vi "Read DO Data Value.vi"(8 "error in (no error)":errorcluster, 9 "Name":string, 10 "DO IOName (enum)":variant, 11 "DAQ":refnum<class "DAQ.lvclass">) -> (0 "error out":errorcluster, 2 "state":bool, 3 "DAQ":refnum<class "DAQ.lvclass">)   [LabVIEW 2017, in "DAQ.lvclass"]
doc: "Developed by Kevin Thompson\nkevin@thompsonengineering.net\n\nCopyright 2018-2020\nThompson Engineering, LLC"
uses:
  DAQ.lvclass
  DAQ.lvclass/DAQ.ctl
  <vilib>/DAQmx/read.llb/DAQmx Read (Digital Bool 1Line 1Point).vi
  Accessors/Get DAQ Settings.vi
  <vilib>/DAQmx/miscellaneous.llb/DAQmx Fill In Error Info.vi
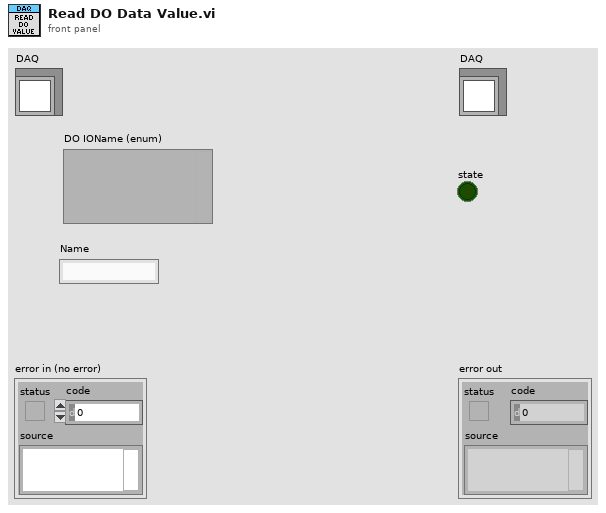
[diagram p1: front panel]
types:
  T1 = typedef "DAQ.lvclass/TD DAQ Settings--cluster.ctl" = cluster{"Simulate DAQ":bool, "DI Settings":T2[], "AI Settings":T3[], "Relay IONames":string[], "AO IONames":string[], "AO NChan SingleTask":bool}
  T2 = typedef "DAQ.lvclass/TD DI Instrument Settings--cluster.ctl" = cluster{"Disable":bool, "DI TaskName":string, "DI RefreshIntv":i32}
  T3 = typedef "DAQ.lvclass/TD AI Instrument Settings--cluster.ctl" = cluster{"Disable":bool, "AI TaskName":string, "AI InstSettings":T4, "SimAI Ranges":T5}
  T4 = typedef "DAQ.lvclass/TD AI InstSettings--cluster.ctl" = cluster{"DaqRate":dbl, "NumSamples":i32}
  T5 = typedef "DAQ.lvclass/TD SimAI Ranges--cluster.ctl" = cluster{"lo":dbl, "hi":dbl}
  T6 = typedef "DAQ.lvclass/TD DO Channel--cluster.ctl" = cluster{"DevName":string, "IOName":string, "IOPath":string, "SchemName":string, "logic":enum16{"Lo", "Hi"}, "DAQmx Task":refnum<k21>}
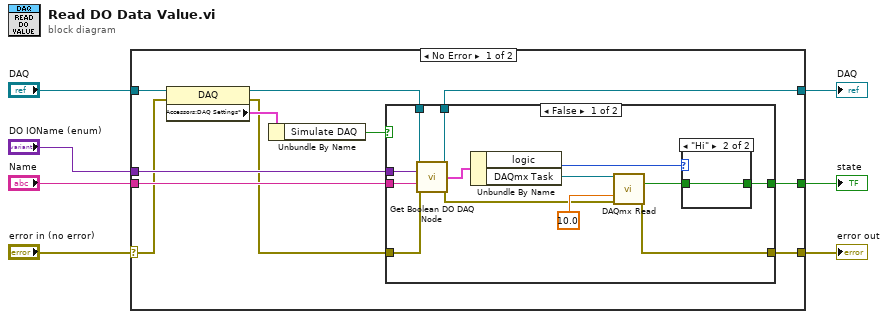
[diagram p0: block diagram]
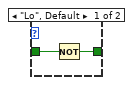
[diagram p2: hidden frame]
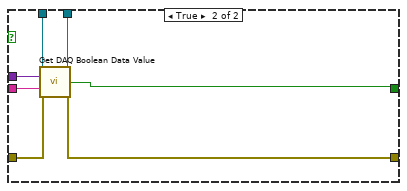
[diagram p3: hidden frame]
diagram:
  n1 = case shown="No Error" "error in (no error)" {
    selector: "error in (no error)" -> [w11 w43]
    tunnel: [w15 w43] -> w6
    tunnel: [w18 w42] -> w4
    tunnel: "DAQ" -> [w12 w42]
    tunnel: "Name" -> [w17 _]
    tunnel: "DO IOName (enum)" -> [w16 _]
    tunnel: [w14 _] -> w1
    frame No Error {
      n2 = property class="DAQ"(reference=w12, error in=w11) -> (reference out=w8:refnum<class "DAQ.lvclass">, error out=w9:errorcluster, "Accessors:DAQ Settings*"=w10:T1)
      n3 = Unbundle By Name(w10) -> ("Simulate DAQ"=w13:bool)
      n4 = case shown="False" w13 {
        tunnel: [w31 w38] -> w18
        tunnel: w17 -> [w30 w41]
        tunnel: w16 -> [w29 w40]
        tunnel: [w20 w36] -> w15
        tunnel: [w28 w35] -> w14
        tunnel: w8 -> [w27 w39]
        tunnel: w9 -> [w19 w37]
        frame False {
          n5 = call "Get Boolean DO DAQ Node.vi"("DAQ"=w27, "IOName (enum)"=w29, "Name"=w30, "error in (no error)"=w19) -> ("DAQ"=w31:refnum<class "DAQ.lvclass">, "DO DAQNode out"=w26:T6, "error out"=w23:errorcluster)  [unwired: 9 in]
          n6 = Unbundle By Name(w26) -> ("logic"=w21:enum16{"Lo", "Hi"}, "DAQmx Task"=w25:refnum<k21>)
          n7 = call-poly <vilib>:"DAQmx Read.vi"("task/channels in"=w25, "timeout"=10.0, "error in"=w23) -> ("data"=w22:bool, "error out"=w20:errorcluster)  [unwired: 10 in, 1 out]
          n8 = case shown="\"Hi\"" w21 {
            tunnel: w22 -> [w33 w34]
            tunnel: [w32 w34] -> w28
            frame "Lo", Default {
              n9 = Not(x=w33) -> (.not. x?=w32:bool)
            }
            frame "Hi" {
            }
          }
        }
        frame True {
          n10 = call "Get DAQ Boolean Data Value.vi"("DAQ"=w39, "IOName (enum)"=w40, "Name"=w41, "error in (no error)"=w37) -> ("DAQ"=w38:refnum<class "DAQ.lvclass">, "Value"=w35:bool, "error out"=w36:errorcluster)  [unwired: 9 in]
        }
      }
    }
    frame Error {
    }
  }
  "error out" <- w6
  "DAQ" <- w4
  "state" <- w1
